vi "Stage Global Variables.vi"() -> ()   [LabVIEW 2014]
uses:
  General/Controls/TableStageModels.ctl
panel:
  in  "Stage Types":cluster{"X":T1, "Y":T1, "Z":T1}
  out "Status":bool[](array[boolean])
  in  "Comm Parameters":variant[](array[variant])
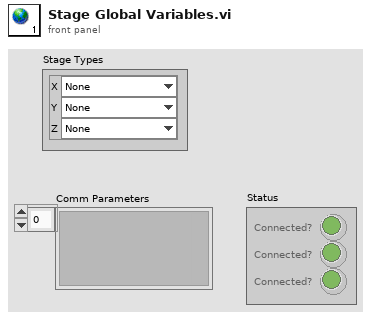
[diagram p1: front panel]
types:
  T1 = typedef "TableStageModels.ctl" = enum16{"None", "CONEX-CC", "Thorlabs LTS"}
diagram:
